vi "NewTemplate.CreateRequests.vi"(8 "error in (no error)":errorcluster) -> (0 "error out":errorcluster, 3 "Requests":T1)   [LabVIEW 2024, in "NewTemplate.lvclass"]
uses:
  NewTemplate.lvclass
  Request Events--cluster.ctl
  Do Something Args.ctl
  JQMHCore/Module/Reply.ctl
  NewTemplate.lvclass/NewTemplate.ctl
  JQMHCore/Module/RQMHModule.lvclass
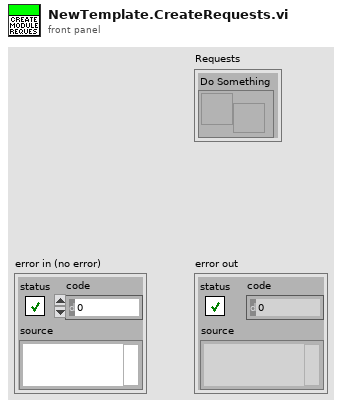
[diagram p1: front panel]
types:
  T1 = typedef "NewTemplate.lvclass/Request Events--cluster.ctl" = cluster{"Do Something":refnum<user-event>}
  T2 = typedef "NewTemplate.lvclass/Do Something Args.ctl" = cluster{"Msg":string}
  T3 = typedef "RQMHModule.lvclass/Reply.ctl" = cluster{"Expects Reply":bool, "Reply":refnum<notifier>}
  T4 = cluster{"Do Something Args":T2, "Reply Payload":T3}
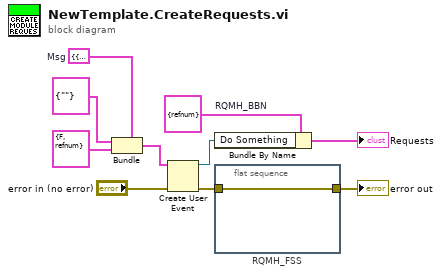
[diagram p0: block diagram]
diagram:
  w4 = T4 {"Do Something Args"={"Msg"=""}, "Reply Payload"={"Expects Reply"=FALSE, "Reply"=refnum}}  # Msg
  n1 = Bundle(cluster=w4, "Do Something Args"=T2 {"Msg"=""}, "Reply Payload"=T3 {"Expects Reply"=FALSE, "Reply"=refnum}) -> (w7:T4)
  n2 = Create User Event(user event datatype=w7, error in="error in (no error)") -> (user event=w3:refnum<user-event>, error out=w1:errorcluster)
  n3 = Bundle By Name "RQMH_BBN"(cluster=T1 {"Do Something"=refnum} ("Requests"), "Do Something"=w3) -> (→"Requests":T1)
  n4 = flat-sequence "RQMH_FSS" {
    tunnel: [w11] -> w2
    tunnel: w1 -> [w11]
    frame #0 {
    }
  }
  "error out" <- w2
